vi "LogError.vi"(0 "Error Map":T1(c390), 2 "LastReportedError":errorcluster, 5 "error in":errorcluster) -> (19 "error out":errorcluster)   [LabVIEW 2019, in "Error handler.lvclass"]
uses:
  Error handler.lvclass
  <vilib>/Utility/SystemLogging/NI_SystemLogging.lvlib
  ErrorLogFile_class/ErrorLogFile.lvclass
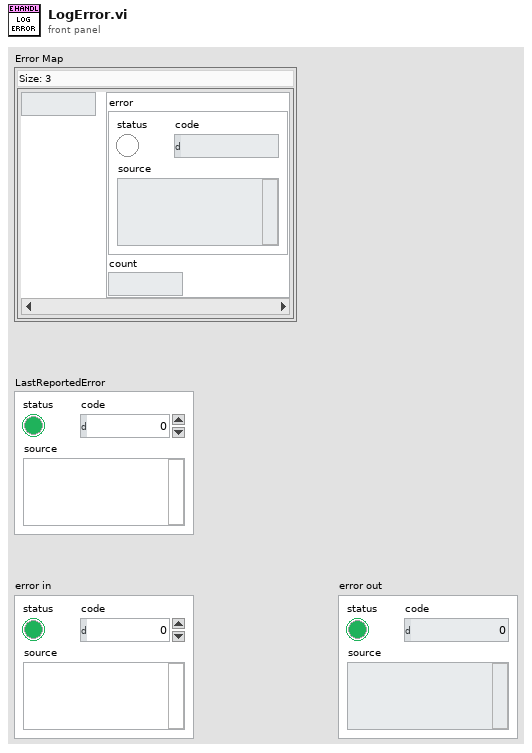
[diagram p1: front panel]
types:
  T1 = map{i32, cluster{"error":errorcluster, "count":i32}}
  T2 = typedef "Error handler.lvclass/ObjectAttributes.ctl" = cluster{"ErrorBroadcastEvent":refnum<user-event>, "LoadFPOnError":bool, "ErrorLogFile":refnum<class "ErrorLogFile.lvclass">, "Testing":bool, "Name":string}
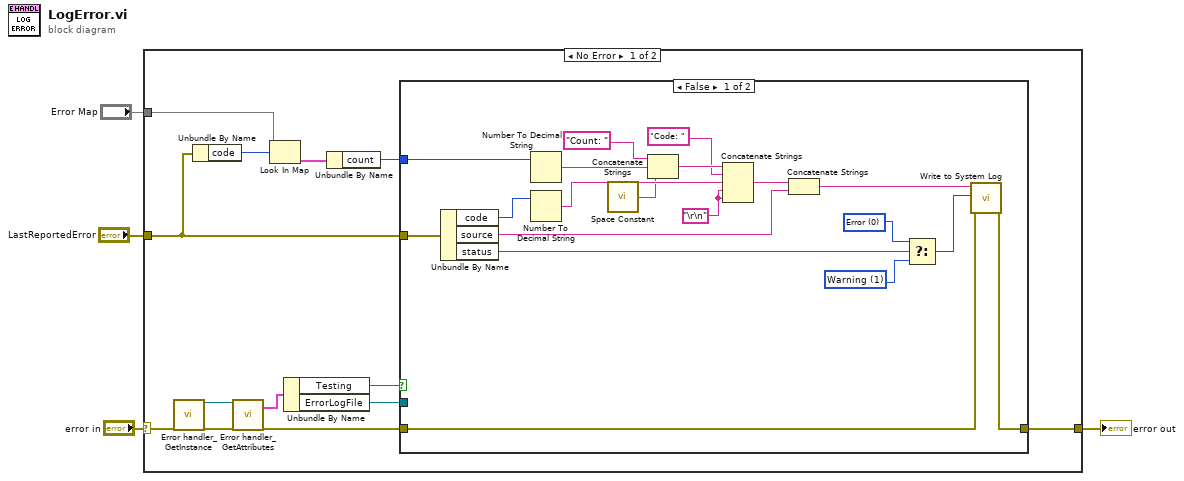
[diagram p0: block diagram]
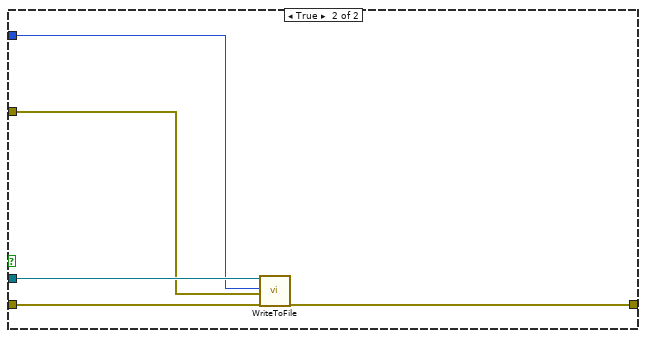
[diagram p2: hidden frame]
diagram:
  n1 = case shown="No Error" "error in" {
    selector: "error in" -> [w12 w42]
    tunnel: [w15 w42] -> w3
    tunnel: "LastReportedError" -> [w6 _]
    tunnel: "Error Map" -> [w17 _]
    frame No Error {
      n2 = call "Error handler_GetInstance.vi"("error in"=w12) -> ("reference out"=w13:refnum<class "Error handler.lvclass">, "error out"=w11:errorcluster)  [unwired: 14 in, 3 out]
      n3 = Unbundle By Name(w6) -> ("code"=w14:i32)
      n4 = call "Error handler_GetAttributes.vi"("reference in"=w13, "error in (no error)"=w11) -> ("Data"=w10:T2, "error out"=w5:errorcluster)  [unwired: 14 in, 2 out]
      n5 = Look In Map(map=w17, key=w14) -> (value=w16:cluster{"error":errorcluster, "count":i32})  [unwired: 1 in, 1 out]
      n6 = Unbundle By Name(w10) -> ("Testing"=w9:bool, "ErrorLogFile"=w8:refnum<class "ErrorLogFile.lvclass">)
      n7 = Unbundle By Name(w16) -> ("count"=w7:i32)
      n8 = case shown="False" w9 {
        tunnel: [w35 w38] -> w15
        tunnel: w7 -> [w23 w37]
        tunnel: w8 -> [_ w41]
        tunnel: w6 -> [w21 w40]
        tunnel: w5 -> [w22 w39]
        frame False {
          w27 = "\r\n"
          w33 = 1 items=["Error", "Warning", "Informational"] ("severity")
          w32 = 0 items=["Error", "Warning", "Informational"] ("severity")
          n9 = Unbundle By Name(w21) -> ("code"=w18:i32, "source"=w19:string, "status"=w20:bool)
          n10 = Number To Decimal String(number=w23) -> (decimal integer string=w36:string)  [unwired: 1 in]
          n11 = Number To Decimal String(number=w18) -> (decimal integer string=w34:string)  [unwired: 1 in]
          n12 = call <vilib>:"Space Constant.vi"() -> ("String"=w24:string)
          n13 = Concatenate Strings("Count: " ("string"), w36, w24) -> (w29:string)
          n14 = Concatenate Strings(w29, "Code: " ("string"), w34, w27, w27) -> (w26:string)
          n15 = Concatenate Strings(w26, w19) -> (w25:string)
          n16 = Select(t=w32, s=w20, f=w33) -> (s? t:f=w31:i32)
          n17 = call <vilib>:"Write to System Log.vi"("error in (no error)"=w22, "severity"=w31, "message"=w25) -> ("error out"=w35:errorcluster)  [unwired: 8 in]
        }
        frame True {
          n18 = call-dynamic "WriteToFile.vi"("object in"=w41, "Count"=w37, "ReportedError"=w40, "Error In"=w39) -> ("Error Out"=w38:errorcluster)  [unwired: 14 in, 1 out]
        }
      }
    }
    frame Error {
    }
  }
  "error out" <- w3
